vi "create.vi"   [LabVIEW 2013, in "call by reference action.lvclass"]
uses:
  call by reference action.lvclass
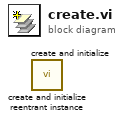
[diagram p0: block diagram]
diagram:
  n1 = call "create and initialize reentrant instance.vi"() -> ()  [unwired: 10 in, 2 out]
  n2 = call "create and initialize.vi"() -> ()  [unwired: 10 in, 2 out]
